vi "readdacsettings.vi"(0 "red":bool, 2 "Path":path, 3 "error in (no error)":errorcluster) -> (5 "Path 2":path, 6 "?":T1, 7 "error out":errorcluster)   [LabVIEW 2012]
uses:
  <vilib>/Utility/config.llb/Read Key (Double).vi
  <vilib>/Utility/config.llb/NI_LVConfig.lvlib
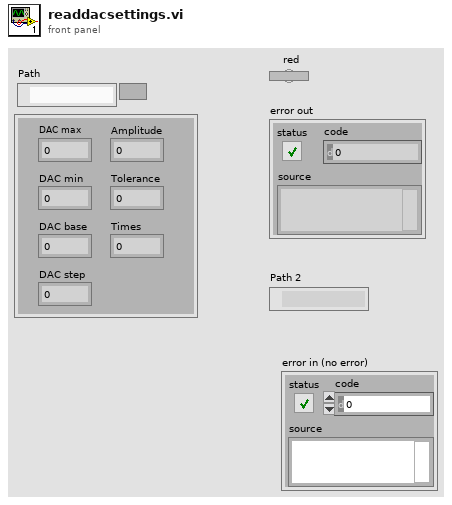
[diagram p1: front panel]
types:
  T1 = cluster{"DAC max":dbl, "DAC min":dbl, "DAC base":dbl, "DAC step":dbl, "Amplitude":dbl, "Tolerance":dbl, "Times":dbl}
  T2 = typedef "NI_LVConfig.lvlib/Config Data RefNum.ctl" = refnum<k1>
  T3 = cluster{"value":dbl, "value":dbl, "value":dbl, "value":dbl, "value":dbl, "value":dbl, "value":dbl}
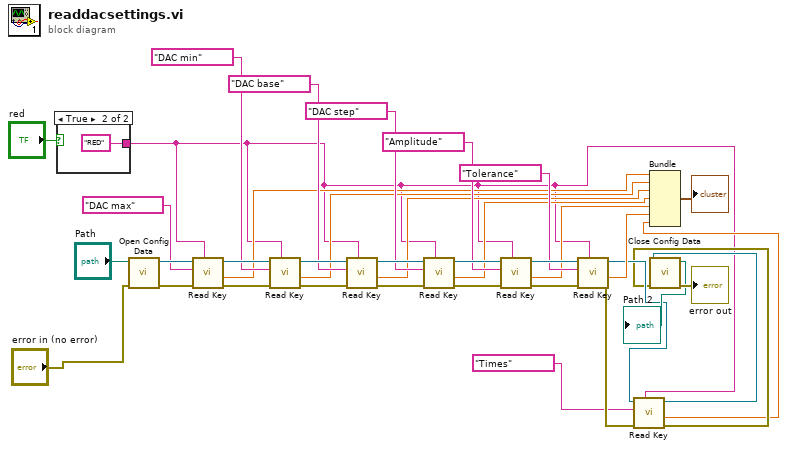
[diagram p0: block diagram]
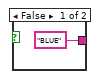
[diagram p2: hidden frame]
diagram:
  n1 = case shown="True" "red" {
    tunnel: ["BLUE" "RED"] -> w3
    frame False {
    }
    frame True {
    }
  }
  n2 = call <vilib>:"Open Config Data.vi"("error in (no error)"="error in (no error)", "configuration file path"="Path") -> ("error out"=w30:errorcluster, "refnum"=w36:T2)  [unwired: 7 in, 1 out]
  n3 = call-poly <vilib>:"Read Key.vi"("section"=w3, "error in (no error)"=w30, "key"="DAC max", "refnum"=w36) -> ("error out"=w29:errorcluster, "value"=w11:dbl, "refnum out"=w35:T2)  [unwired: 4 in, 1 out]
  n4 = call-poly <vilib>:"Read Key.vi"("section"=w3, "error in (no error)"=w29, "key"="DAC min", "refnum"=w35) -> ("error out"=w28:errorcluster, "value"=w12:dbl, "refnum out"=w34:T2)  [unwired: 4 in, 1 out]
  n5 = call-poly <vilib>:"Read Key.vi"("section"=w3, "error in (no error)"=w28, "key"="DAC base", "refnum"=w34) -> ("error out"=w27:errorcluster, "value"=w13:dbl, "refnum out"=w33:T2)  [unwired: 4 in, 1 out]
  n6 = call-poly <vilib>:"Read Key.vi"("section"=w3, "error in (no error)"=w27, "key"="DAC step", "refnum"=w33) -> ("error out"=w26:errorcluster, "value"=w14:dbl, "refnum out"=w32:T2)  [unwired: 4 in, 1 out]
  n7 = call-poly <vilib>:"Read Key.vi"("section"=w3, "error in (no error)"=w26, "key"="Amplitude", "refnum"=w32) -> ("error out"=w25:errorcluster, "value"=w15:dbl, "refnum out"=w31:T2)  [unwired: 4 in, 1 out]
  n8 = call-poly <vilib>:"Read Key.vi"("section"=w3, "error in (no error)"=w25, "key"="Tolerance", "refnum"=w31) -> ("error out"=w7:errorcluster, "value"=w16:dbl, "refnum out"=w8:T2)  [unwired: 4 in, 1 out]
  n9 = call-poly <vilib>:"Read Key.vi"("section"=w3, "error in (no error)"=w7, "key"="Times", "refnum"=w8) -> ("error out"=w5:errorcluster, "value"=w4:dbl, "refnum out"=w6:T2)  [unwired: 4 in, 1 out]
  n10 = Bundle("value"=w11, "value"=w12, "value"=w13, "value"=w14, "value"=w15, "value"=w16, "value"=w4) -> (→"?":T3)  [unwired: 1 in]
  n11 = call <vilib>:"Close Config Data.vi"("error in (no error)"=w5, "refnum"=w6) -> ("error out"=→"error out":errorcluster, "file path"=→"Path 2":path)  [unwired: 8 in]
